vi "ReadGetFoodQuantity.vi"(8 "error in (no error)":errorcluster, 11 "Cat in":refnum<class "Cat.lvclass">) -> (0 "error out":errorcluster, 2 "GetFoodQuantity":i32, 3 "Cat out":refnum<class "Cat.lvclass">)   [LabVIEW 2013, in "Cat.lvclass"]
uses:
  Cat.lvclass
  Cat.lvclass/Cat.ctl
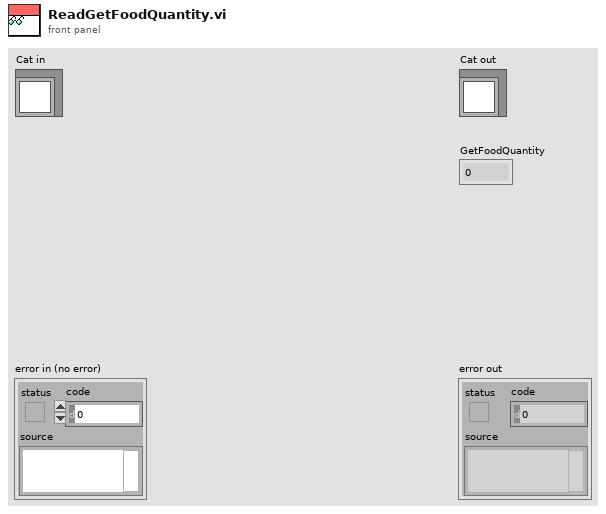
[diagram p1: front panel]
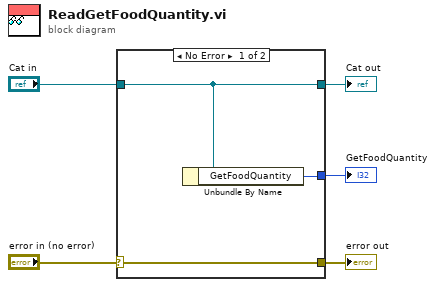
[diagram p0: block diagram]
diagram:
  n1 = case shown="No Error" "error in (no error)" {
    selector: "error in (no error)" -> [w8 w9]
    tunnel: [w8 w9] -> w4
    tunnel: [w6 w10] -> w2
    tunnel: "Cat in" -> [w6 w10]
    tunnel: [w7 _] -> w1
    frame No Error {
      n2 = Unbundle By Name(w6) -> ("GetFoodQuantity"=w7:i32)
    }
    frame Error {
    }
  }
  "error out" <- w4
  "Cat out" <- w2
  "GetFoodQuantity" <- w1
